vi "programacion examen de las 5 y20.vi"() -> ()   [LabVIEW 2011]
panel:
  out "Temperatura mayor":dbl
  out "Temperatura promedio":dbl
  out "61-100":bool
  out "31-60":bool
  out "1-30":bool
  out "Thermometer":i32(slide) scale=0.0..100.0
  # "Generar la temperatura entre 1-100 el\nprograma se detiene cuando la temperatura \nes mayor a 90.\nAl final debera presentar la temp promedio \ndurante el programa se ejecute debera de encender\nlos led de acuerdo al rango.\nobtener la temperatura mayor."
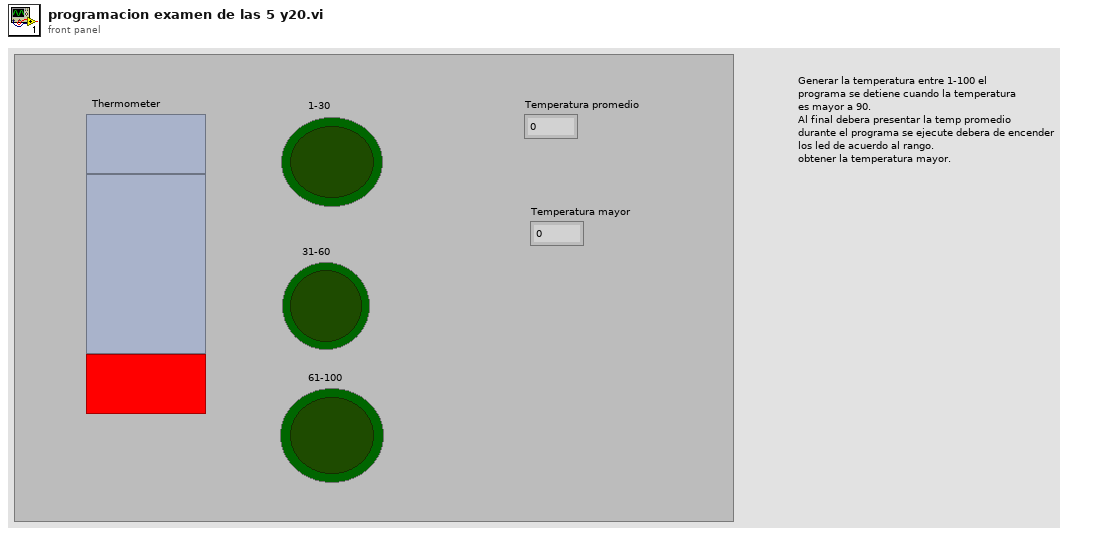
[diagram p1: front panel]
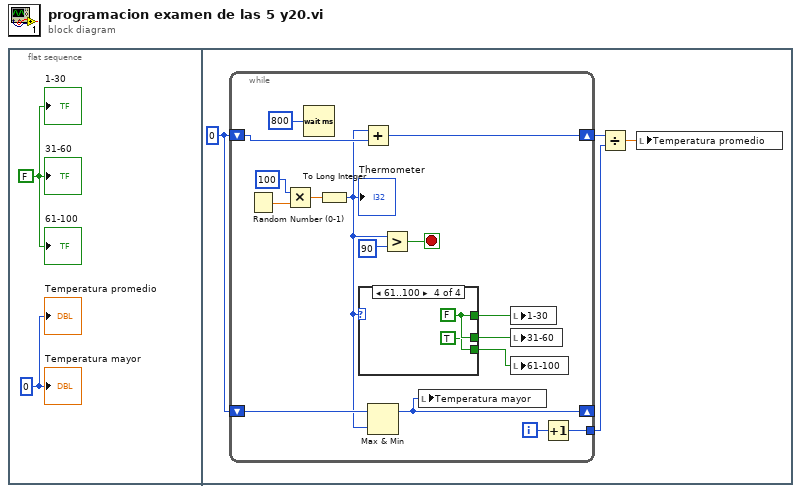
[diagram p0: block diagram]
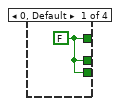
[diagram p2: hidden frame]
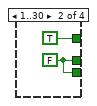
[diagram p3: hidden frame]
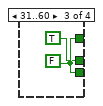
[diagram p4: hidden frame]
diagram:
  n1 = flat-sequence {
    frame #0 {
      w1 = FALSE
      w2 = 0
      "Temperatura promedio" <- w2
      "Temperatura mayor" <- w2
      "1-30" <- w1
      "61-100" <- w1
      "31-60" <- w1
    }
    frame #1 {
      w6 = 0
      n2 = while {
        tunnel: [w13] -> w5
        shift-right: [w11] -> w4
        shift-left: w6 -> [w12]
        shift-right: [w7] -> _
        shift-left: w6 -> [w9]
        i -> [w17]
        stop <- w21 stop-if-true
        n3 = Random Number (0-1)() -> (number: 0 to 1=w19:dbl)
        n4 = Multiply(x=100, y=w19) -> (x*y=w18:dbl)
        n5 = Wait (ms)(milliseconds to wait=u32 800) -> ()  [unwired: 1 out]
        n6 = To Long Integer(number=w18) -> (32bit integer=w8:i32)
        "Thermometer" <- w8
        n7 = case shown="61..100" w8 {
          tunnel: [w23 TRUE w27 w29] -> w16
          tunnel: [w23 w24 TRUE w29] -> w15
          tunnel: [w23 w24 w27 TRUE] -> w14
          frame 0, Default {
            w23 = FALSE
          }
          frame 1..30 {
            w24 = FALSE
          }
          frame 31..60 {
            w27 = FALSE
          }
          frame 61..100 {
            w29 = FALSE
          }
        }
        n8 = Add(x=w8, y=w12) -> (x+y=w11:i32)
        n9 = Max & Min(x=w9, y=w8) -> (max(x,y)=w7:i32)  [unwired: 1 out]
        n10 = Greater?(x=w8, y=90) -> (0:w21:bool)
        n11 = local write "Temperatura mayor"(w7) -> ()
        n12 = local write "1-30"(w16) -> ()
        n13 = local write "31-60"(w15) -> ()
        n14 = local write "61-100"(w14) -> ()
        n15 = Increment(x=w17) -> (x+1=w13:i32)
      }
      n16 = Divide(x=w4, y=w5) -> (x/y=w3:dbl)
      n17 = local write "Temperatura promedio"(w3) -> ()
    }
  }
